vi "ModifyColor.vi"(11 "ControlRefsIn":T1) -> (3 "ControlRefsOut":T1)   [LabVIEW 2013]
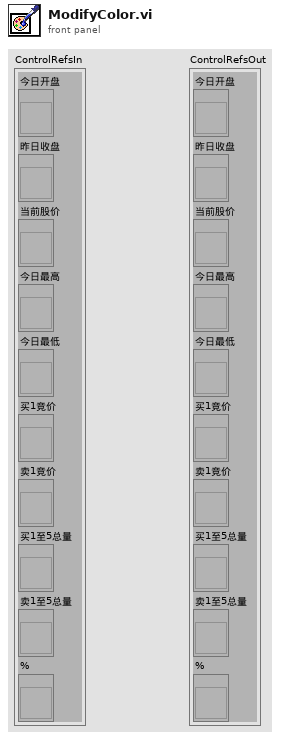
[diagram p1: front panel]
types:
  T1 = cluster{"今日开盘":refnum<vi>, "昨日收盘":refnum<vi>, "当前股价":refnum<vi>, "今日最高":refnum<vi>, "今日最低":refnum<vi>, "买1竞价":refnum<vi>, "卖1竞价":refnum<vi>, "买1至5总量":refnum<vi>, "卖1至5总量":refnum<vi>, "%":refnum<vi>}
  T2 = cluster{"[0]":refnum<vi>, "[1]":refnum<vi>, "[2]":refnum<vi>, "[3]":refnum<vi>, "[4]":refnum<vi>, "[5]":refnum<vi>, "[6]":refnum<vi>, "[7]":refnum<vi>, "[8]":refnum<vi>, "[9]":refnum<vi>}
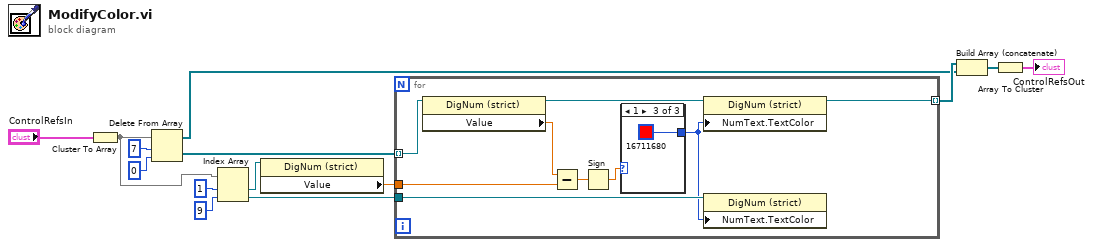
[diagram p0: block diagram]
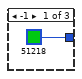
[diagram p2: hidden frame]
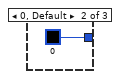
[diagram p3: hidden frame]
diagram:
  n1 = Cluster To Array(cluster="ControlRefsIn") -> (array=w1:refnum<vi>[])
  n2 = Delete From Array(array=w1, length=7, index=0) -> (deleted portion=w2:refnum<vi>[], array with subset deleted=w3:refnum<vi>[])
  n3 = Index Array(array=w1, index #1=1 ("index"), index #2=9 ("index")) -> (element #1=w12:refnum<vi>, element #2=w4:refnum<vi>)
  n4 = property class="DigNum (strict)"(reference=w12) -> ("Value"=w11:dbl)  [unwired: 1 in, 2 out]
  n5 = for {
    tunnel: w2 -> [w23] mode=indexing
    tunnel: w11 -> [w21]
    tunnel: [w17] -> w6 mode=indexing
    tunnel: w4 -> [w16]
    n6 = property class="DigNum (strict)"(reference=w23) -> (reference out=w18:refnum<vi>, "Value"=w22:dbl)  [unwired: 1 in, 1 out]
    n7 = Subtract(x=w22, y=w21) -> (x-y=w20:dbl)
    n8 = Sign(1:w20) -> (0:w19:dbl)
    n9 = case shown="1" w19 {
      tunnel: [u32 51218 u32 0 u32 16711680] -> w15
      frame -1 {
      }
      frame 0, Default {
      }
      frame 1 {
      }
    }
    n10 = property class="DigNum (strict)"(reference=w18, "NumText.TextColor"=w15) -> (reference out=w17:refnum<vi>)  [unwired: 1 in, 1 out]
    n11 = property class="DigNum (strict)"(reference=w16, "NumText.TextColor"=w15) -> ()  [unwired: 1 in, 2 out]
  }
  n12 = Build Array (concatenate)(w6, w3) -> (w5:refnum<vi>[])
  n13 = Array To Cluster(array=w5) -> (cluster=→"ControlRefsOut":T2)
